vi "Get Event Timing Measurements.vi"(7 "return not-added measurements (T)":bool=TRUE, 8 "error in (no error)":errorcluster, 11 "Item Ref in":T1 format="%.0x") -> (0 "error out":errorcluster, 1 "measurements refs":T1[](array[typedef]) format="%.0x", 2 "measurements":T2[](array[typedef]), 3 "Item Ref out":T1 format="%.0x", 5 "not present indexes":i32[](array[numeric]))   [LabVIEW 2015, in "Engine Simulation Toolkit System Explorer.lvlib"]
uses:
  Engine Simulation Toolkit System Explorer.lvlib
  Event Timing Measurement.ctl
  Polarity.ctl
  <vilib>/NI Veristand/Custom Device API/Custom Device Item Ref.ctl
  Shared/Properties.vi
  <vilib>/NI Veristand/Custom Device API/Get Item Property (String).vi
  Shared/Constants and GUIDs.vi
  <vilib>/NI Veristand/Custom Device API/Get Item Property (U16).vi
  Shared/Engine Simulation Toolkit Shared.lvlib
  <vilib>/NI Veristand/Custom Device API/Custom Device API.lvlib
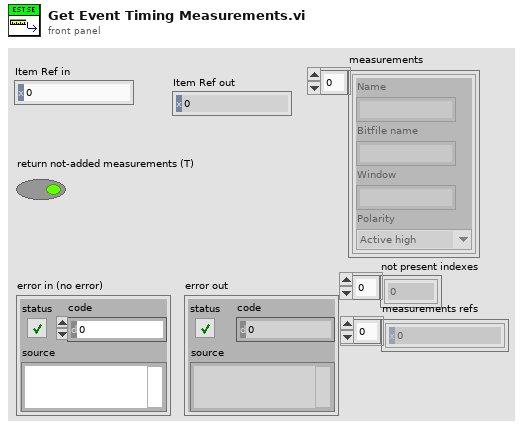
[diagram p1: front panel]
types:
  T1 = typedef "Custom Device API.lvlib/Custom Device Item Ref.ctl" = u64
  T2 = typedef "Engine Simulation Toolkit System Explorer.lvlib/Event Timing Measurement.ctl" = cluster{"Name":string, "Bitfile name":string, "Window":string, "Polarity":T3}
  T3 = typedef "Engine Simulation Toolkit System Explorer.lvlib/Polarity.ctl" = enum16{"Active low", "Active high"}
  T4 = typedef "Custom Device API.lvlib/Custom Device Item Info.ctl" = cluster{"Name":string, "Is Channel":bool, "GUID":string, "Is Waveform":bool}
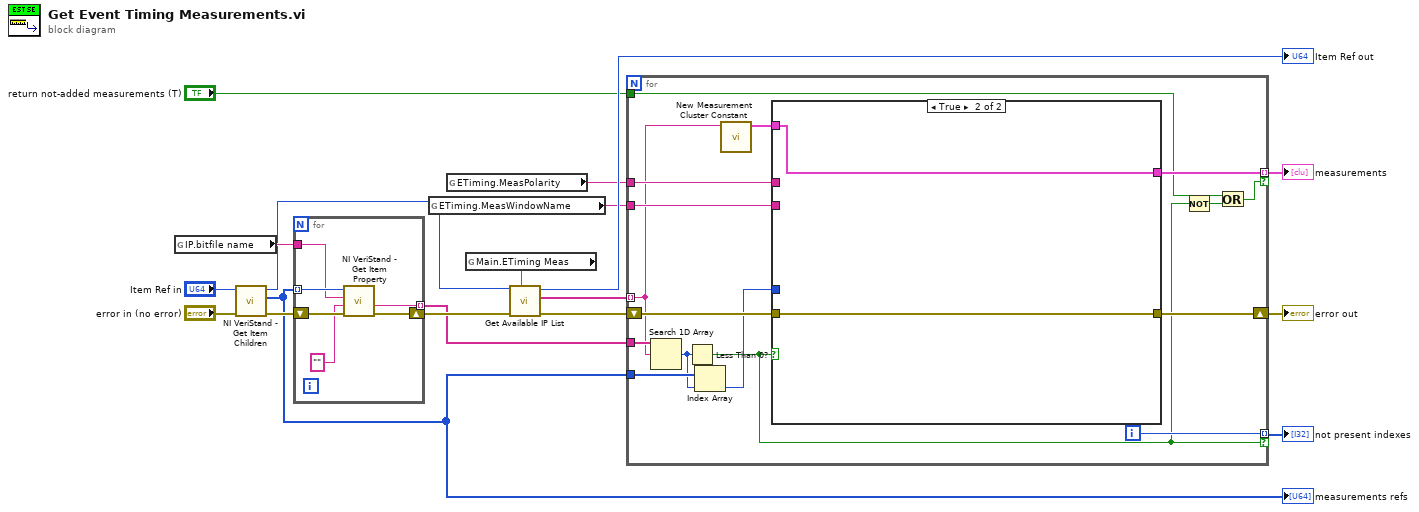
[diagram p0: block diagram]
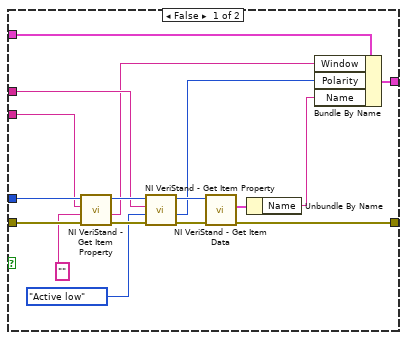
[diagram p2: hidden frame]
diagram:
  n1 = global read "Properties.vi" "IP.bitfile name"() -> (w6:string)
  n2 = call <vilib>:"NI VeriStand - Get Item Children.vi"("error in (no error)"="error in (no error)", "Item Ref in"="Item Ref in") -> ("error out"=w7:errorcluster, "Child Refs"=w2:T1[], "Item Ref out"=w5:T1)  [unwired: 6 in, 1 out]
  "measurements refs" <- w2
  n3 = for {
    shift-right: [w21] -> w4
    shift-left: w7 -> [w24]
    tunnel: w2 -> [w23] mode=indexing
    tunnel: w6 -> [w22]
    tunnel: [w19] -> w3 mode=indexing
    n4 = call-poly <vilib>:"NI VeriStand - Get Item Property.vi"("error in (no error)"=w24, "Default Value"="", "Property Name"=w22, "Item Ref in"=w23) -> ("error out"=w21:errorcluster, "Value"=w19:string)  [unwired: 4 in, 2 out]
  }
  n5 = global read "Properties.vi" "ETiming.MeasWindowName"() -> (w11:string)
  n6 = global read "Properties.vi" "ETiming.MeasPolarity"() -> (w10:string)
  n7 = global read "Properties.vi" "Main.ETiming Meas"() -> (w17:string)
  n8 = call "Get Available IP List.vi"("ip list property name"=w17, "error in (no error)"=w4, "Item Ref in"=w5) -> ("error out"=w15:errorcluster, "ips available"=w14:string[], "Item Ref out"=→"Item Ref out":T1)  [unwired: 6 in]
  n9 = for {
    tunnel: [w29] -> w18 mode=indexing if=w27
    shift-right: [w38] -> w12
    shift-left: w15 -> [w36]
    tunnel: w14 -> [w30] mode=indexing
    tunnel: w11 -> [w40]
    tunnel: w10 -> [w39]
    tunnel: [w37] -> w9 mode=indexing if=w28
    tunnel: w3 -> [w35]
    tunnel: w2 -> [w34]
    tunnel: "return not-added measurements (T)" -> [w26]
    i -> [w37]
    n10 = Search 1D Array(1D array=w35, element=w30) -> (index of element=w33:i32)  [unwired: 1 in]
    n11 = Less Than 0?(x=w33) -> (x < 0?=w28:bool)
    n12 = Index Array(array=w34, index=w33) -> (element=w32:T1)
    n13 = call "New Measurement Cluster Constant.vi"("Bitfile name"=w30) -> ("Measurement"=w31:T2)  [unwired: 10 in]
    n14 = case shown="True" w28 {
      tunnel: w36 -> [w57 w59]
      tunnel: w32 -> [w56 _]
      tunnel: w40 -> [w55 _]
      tunnel: w39 -> [w52 _]
      tunnel: [w50 w59] -> w38
      tunnel: w31 -> [w45 w58]
      tunnel: [w41 w58] -> w29
      frame False {
        n15 = call-poly <vilib>:"NI VeriStand - Get Item Property.vi"("error in (no error)"=w57, "Default Value"="", "Property Name"=w55, "Item Ref in"=w56) -> ("error out"=w54:errorcluster, "Value"=w44:string, "Item Ref out"=w53:T1)  [unwired: 4 in, 1 out]
        n16 = call-poly <vilib>:"NI VeriStand - Get Item Property.vi"("error in (no error)"=w54, "Default Value"=Polarity."Active low" ("Polarity"), "Property Name"=w52, "Item Ref in"=w53) -> ("error out"=w51:errorcluster, "Value"=w43:u16, "Item Ref out"=w46:T1)  [unwired: 4 in, 1 out]
        n17 = call <vilib>:"NI VeriStand - Get Item Data.vi"("error in (no error)"=w51, "Item Ref in"=w46) -> ("error out"=w50:errorcluster, "Item Info"=w49:T4)  [unwired: 6 in, 2 out]
        n18 = Unbundle By Name(w49) -> ("Name"=w42:string)
        n19 = Bundle By Name(cluster=w45, "Window"=w44, "Polarity"=w43, "Name"=w42) -> (w41:T2)
      }
      frame True {
      }
    }
    n20 = Not(x=w28) -> (.not. x?=w25:bool)
    n21 = Or(x=w26, y=w25) -> (x .or. y?=w27:bool)
  }
  "error out" <- w12
  "measurements" <- w18
  "not present indexes" <- w9
